vi "AuMT8852B SCO Connect - Disconnect.vi"(5 "Connect / Disconnect (Connect)":enum16{"Disconnect", "Connect"}(ring)=enum."Connect", 7 "Channel (1)":i32=1, 8 "error in (no error)":errorcluster, 11 "VISA session":refnum<visa-resource-name>) -> (0 "error out":errorcluster, 2 "error code":i32, 3 "VISA session out":refnum<visa-resource-name>)   [LabVIEW 2017]
doc: "Anritsu MT8852B Bluetooth Tester\n\nThis command is used to create or terminate a SCO connection on the specified channel. When the operation has been completed, the SCC bit in the CHG register will be set. The current state of the SCO connections can be obtained by using the STATUS command (Instrument Status Query).\n\nINPUTS\nChannel - Which SCO channel (1-3) will be affected.\nConnect / Disconnect - operation to perform on the selected channel."
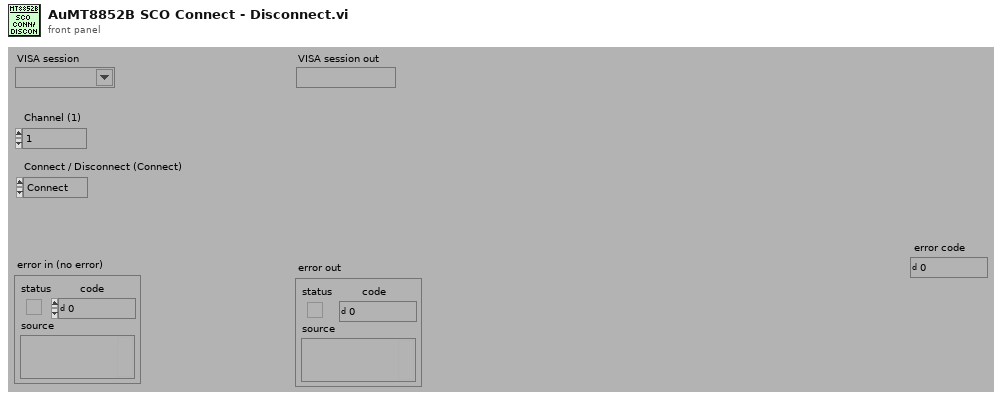
[diagram p1: front panel]
types:
  T1 = enum16{"Simulate", "Range check", "Cache", "Query instrument status"}
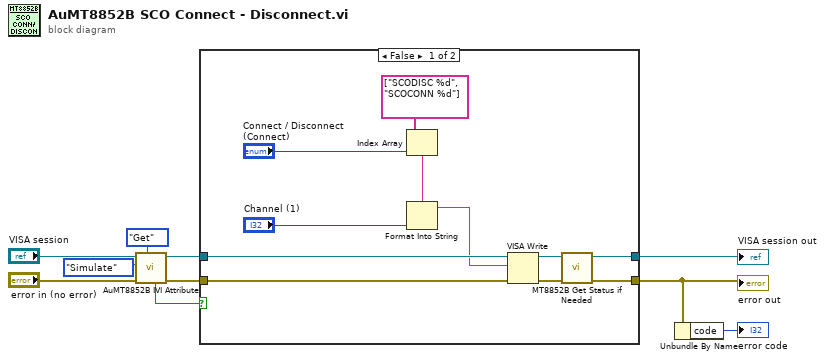
[diagram p0: block diagram]
diagram:
  n1 = call <instrlib>:"AuMT8852B IVI Attribute.vi"("Set/Get (Set)"=enum16{"Set", "Get"}."Get", "error in (no error)"="error in (no error)", "Flag (Simulate)"=T1."Simulate", "VISA session"="VISA session") -> ("error out"=w9:errorcluster, "VISA session out"=w10:refnum<visa-resource-name>, "Value out"=w6:bool)  [unwired: 5 in]
  n2 = case shown="False" w6 {
    tunnel: [w12 w22] -> w1
    tunnel: [w13 w23] -> w5
    tunnel: w10 -> [w21 w23]
    tunnel: w9 -> [w20 w22]
    frame False {
      n3 = Index Array(array=string[] ["SCODISC %d", "SCOCONN %d"], index="Connect / Disconnect (Connect)") -> (element=w14:string)
      n4 = Format Into String(format string=w14, "Channel (1)") -> (resulting string=w17:string)  [unwired: 2 in, 1 out]
      n5 = VISA Write(VISA resource name=w21, write buffer=w17, error in (no error)=w20) -> (VISA resource name out=w16:refnum<visa-resource-name>, error out=w19:errorcluster)  [unwired: 1 out]
      n6 = call <instrlib>:"MT8852B Get Status if Needed.vi"("error in (no error)"=w19, "VISA session"=w16) -> ("error out"=w12:errorcluster, "VISA session out"=w13:refnum<visa-resource-name>)  [unwired: 8 in]
    }
    frame True {
    }
  }
  "VISA session out" <- w5
  "error out" <- w1
  n7 = Unbundle By Name(w1) -> ("code"=→"error code":i32)
